vi "MarkerData.vi"(0 "VISA IN":refnum<visa-resource-name>, 2 "Marker number":i32=1, 5 "error in":errorcluster, 7 "Channel":i32=1) -> (14 "VISA Out":refnum<visa-resource-name>, 15 "X Axis":dbl, 16 "Y Real":dbl, 18 "Y Imaginary":dbl, 19 "error out":errorcluster)   [LabVIEW 2018, in "PNA-X.lvlib"]
doc: "*Critical Note:\nA measurement must be active prior to using the marker functions."
uses:
  PNA-X.lvlib
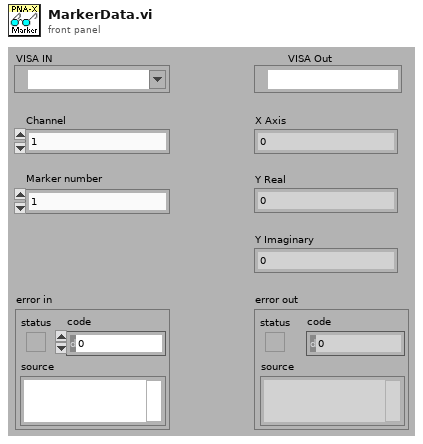
[diagram p1: front panel]
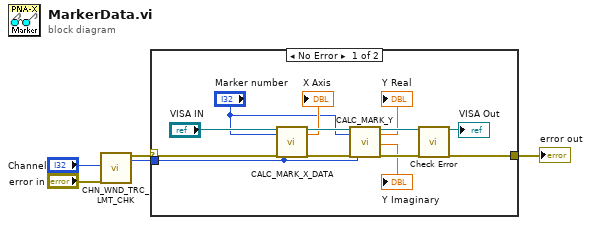
[diagram p0: block diagram]
diagram:
  n1 = call "CHN_WND_TRC_LMT_CHK.vi"("Channel"="Channel", "error in"="error in") -> ("error out"=w1:errorcluster, "Channel"=w2:i32)  [unwired: 13 in, 3 out]
  n2 = case shown="No Error" w1 {
    selector: w1 -> [w9 w20]
    tunnel: [w18 w19] -> w5
    tunnel: w2 -> [w6 _]
    frame No Error {
      n3 = call "CALC_MARK_X_DATA.vi"("VISA IN"="VISA IN", "Marker number"="Marker number", "error in"=w9, "Channel"=w6) -> ("VISA Out"=w14:refnum<visa-resource-name>, "X Axis"=→"X Axis":dbl, "error out"=w13:errorcluster)  [unwired: 13 in]
      n4 = call "CALC_MARK_Y.vi"("VISA IN"=w14, "Marker number"="Marker number", "error in"=w13, "Channel"=w6) -> ("VISA Out"=w15:refnum<visa-resource-name>, "Real"=→"Y Real":dbl, "Imaginary"=→"Y Imaginary":dbl, "error out"=w16:errorcluster)  [unwired: 12 in]
      n5 = call "Check Error.vi"("VISA Resource Name"=w15, "error in (no error)"=w16) -> ("dup VISA session"=→"VISA Out":refnum<visa-resource-name>, "error out"=w18:errorcluster)  [unwired: 16 in]
    }
    frame Error {
      n6 = call <vilib>:"Simple Error Handler.vi"("error in (no error)"=w20) -> ("error out"=w19:errorcluster)  [unwired: 4 in, 4 out]
    }
  }
  "error out" <- w5
